vi "Execute Next Test.vi"(8 "error in (no error)":errorcluster, 11 "Test Manager in":refnum<class "Test Manager.lvclass">) -> (0 "error out":errorcluster, 3 "Test Manager out":refnum<class "Test Manager.lvclass">)   [LabVIEW 2020, in "Test Manager.lvlib" / "Test Manager.lvclass"]
uses:
  Test Manager.lvclass
  Test Manager.lvclass/Test Manager.ctl
  _Abstract Classes/Test/Test.lvclass
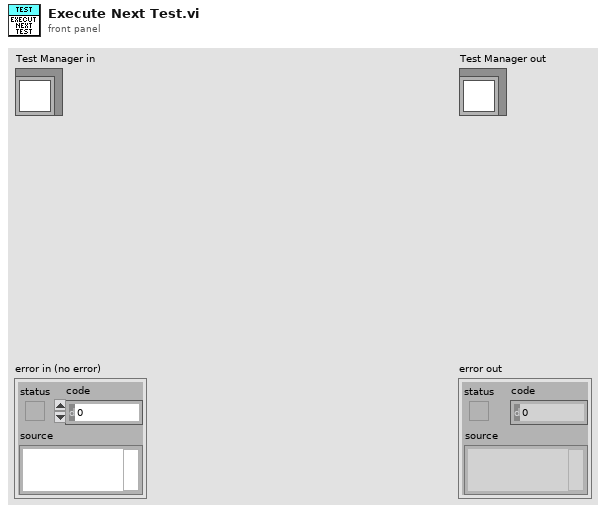
[diagram p1: front panel]
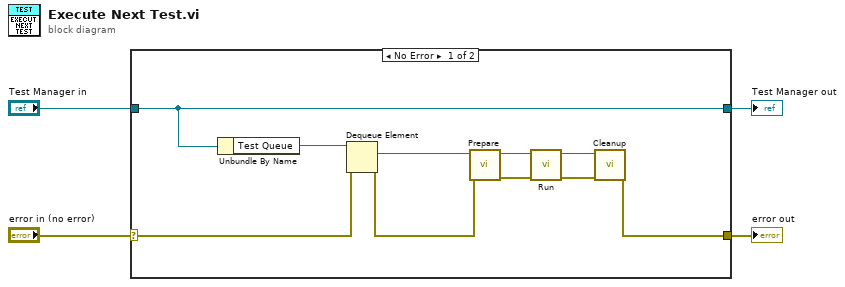
[diagram p0: block diagram]
diagram:
  n1 = case shown="No Error" "error in (no error)" {
    selector: "error in (no error)" -> [w6 w16]
    tunnel: [w8 w16] -> w3
    tunnel: [w14 w15] -> w1
    tunnel: "Test Manager in" -> [w14 w15]
    frame No Error {
      n2 = Unbundle By Name(w14) -> ("Test Queue"=w13:refnum<queue>)
      n3 = Dequeue Element(queue=w13, error in (no error)=w6) -> (element=w7:refnum<class "Test.lvclass">, error out=w5:errorcluster)  [unwired: 1 in, 2 out]
      n4 = call-dynamic "Prepare.vi"("error in (no error)"=w5, "Test in"=w7) -> ("error out"=w10:errorcluster, "Test out"=w12:refnum<class "Test.lvclass">)  [unwired: 8 in]
      n5 = call-dynamic "Run.vi"("error in (no error)"=w10, "Test in"=w12) -> ("error out"=w9:errorcluster, "Test out"=w11:refnum<class "Test.lvclass">)  [unwired: 8 in]
      n6 = call-dynamic "Cleanup.vi"("error in (no error)"=w9, "Test in"=w11) -> ("error out"=w8:errorcluster)  [unwired: 8 in, 1 out]
    }
    frame Error {
    }
  }
  "error out" <- w3
  "Test Manager out" <- w1
